vi "Action.vi"(8 "error in (no error)":errorcluster, 10 "Actor in":refnum<class "Tamagotchi Basic Actor.lvclass">, 11 "Spaghetti Message in":refnum<class "Spaghetti Message.lvclass">) -> (0 "error out":errorcluster, 2 "Actor out":refnum<class "Tamagotchi Basic Actor.lvclass">, 3 "Spaghetti Message out":refnum<class "Spaghetti Message.lvclass">)   [LabVIEW 2026, in "Spaghetti Message.lvclass"]
uses:
  Spaghetti Message.lvclass
  Tamagotchi Basic Actor/Tamagotchi Basic Actor.lvclass
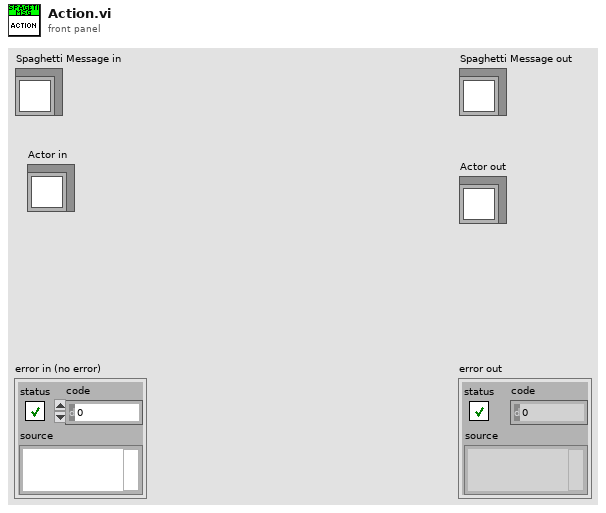
[diagram p1: front panel]
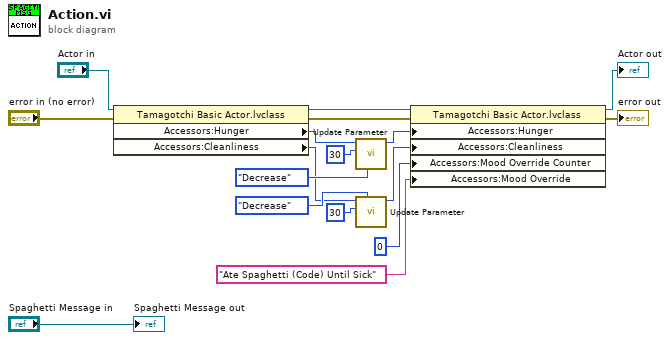
[diagram p0: block diagram]
diagram:
  n1 = property class="Tamagotchi Basic Actor.lvclass"(reference="Actor in", error in="error in (no error)") -> (reference out=w15:refnum<class "Tamagotchi Basic Actor.lvclass">, error out=w2:errorcluster, "Accessors:Hunger"=w9:i16, "Accessors:Cleanliness"=w8:i16)
  n2 = call "Update Parameter.vi"("Action"=enum16{"Increase", "Decrease"}."Decrease", "Modifier"=i16 30 ("y"), "Parameter"=w9) -> ("New Value"=w7:i16)  [unwired: 8 in]
  n3 = call "Update Parameter.vi"("Action"=enum16{"Increase", "Decrease"}."Decrease", "Modifier"=i16 30 ("y"), "Parameter"=w8) -> ("New Value"=w6:i16)  [unwired: 8 in]
  n4 = property class="Tamagotchi Basic Actor.lvclass"(reference=w15, error in=w2, "Accessors:Hunger"=w7, "Accessors:Cleanliness"=w6, "Accessors:Mood Override Counter"=u32 0 ("Mood Override Counter"), "Accessors:Mood Override"="Ate Spaghetti (Code) Until Sick" ("Mood Override")) -> (reference out=→"Actor out":refnum<class "Tamagotchi Basic Actor.lvclass">, error out=→"error out":errorcluster)
  "Spaghetti Message out" <- "Spaghetti Message in"
